vi "Elevator Controller Code.vi"(5 "Cut Off Switch":bool, 6 "Bottom Switch":bool, 7 "Top Switch":bool, 8 "Down":bool, 9 "Up":bool, 10 "Decrease":bool, 11 "Increase":bool) -> (1 "Tote Offset":dbl, 3 "Motor Value":dbl)   [LabVIEW 2014]
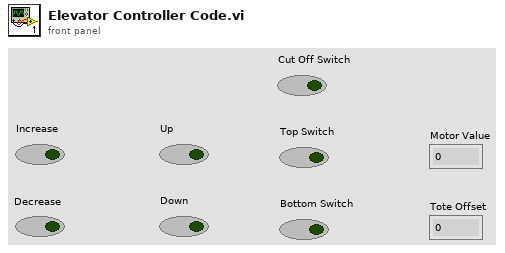
[diagram p1: front panel]
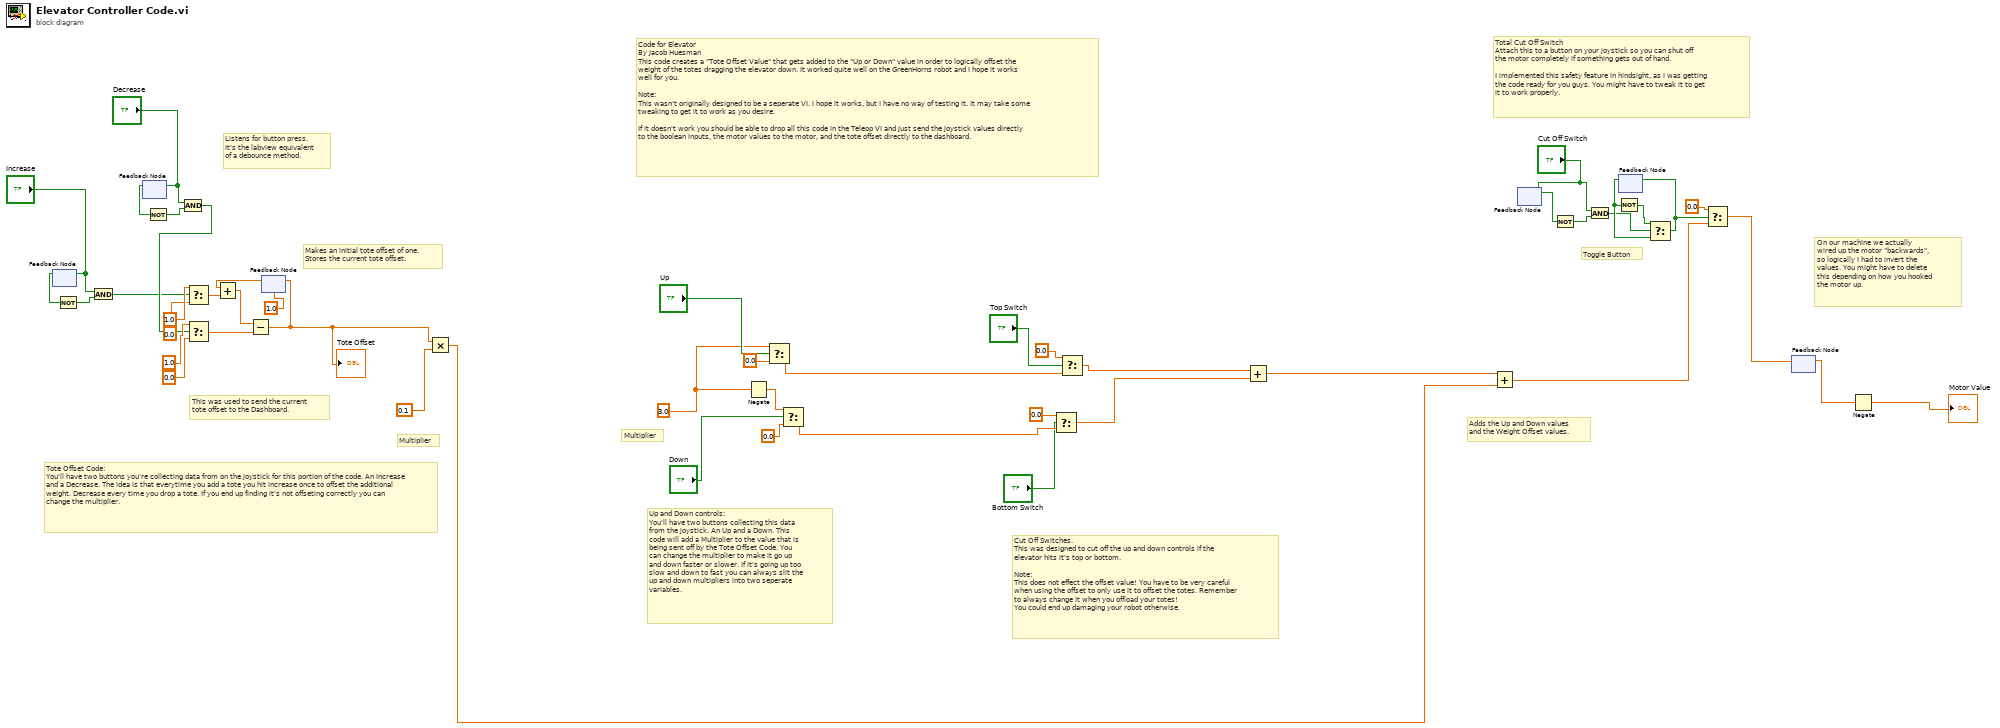
[diagram p0: block diagram]
diagram:
  w18 = 3.0
  # "Toggle Button"
  # "Total Cut Off Switch\nAttach this to a button on your joystick so you can shut off\nthe motor completely if something gets out of hand.\n\nI implemented this safety feature in hindsight, as I was getting\nthe code ready for you guys. You might have to tweak it to get \nit to work properly."
  # "Cut Off Switches.\nThis was designed to cut off the up and down controls if the\nelevator hits it's top or bottom.\n\nNote:\nThis does not effect the offset value! You have to be very careful\nwhen using the offset to only use it to offset the totes. Remember\nto always change it when you offload your totes! \nYou could end up damaging your robot otherwise."
  # "On our machine we actually\nwired up the motor \"backwards\",\nso logically I had to invert the\nvalues. You might have to delete\nthis depending on how you hooked\nthe motor up."
  # "Adds the Up and Down values\nand the Weight Offset values."
  # "Makes an initial tote offset of one.\nStores the current tote offset."
  # "Listens for button press.\nIt's the labview equivalent\nof a debounce method."
  # "This was used to send the current \ntote offset to the Dashboard."
  # "Multiplier"
  # "Up and Down controls:\nYou'll have two buttons collecting this data\nfrom the joystick. An Up and a Down. This \ncode will add a Multiplier to the value that is\nbeing sent off by the Tote Offset Code. You\ncan change the multiplier to make it go up\nand down faster or slower. If it's going up too\nslow and down to fast you can always slit the\nup and down multipliers into two seperate \nvariables."
  # "Multiplier"
  # "Tote Offset Code:\nYou'll have two buttons you're collecting data from on the joystick for this portion of the code. An Increase and a Decrease. The idea is that everytime you add a tote you hit increase once to offset the additional weight. Decrease every time you drop a tote. If you end up finding it's not offseting correctly you can change the multiplier."
  # "Code for Elevator\nBy Jacob Huesman\nThis code creates a \"Tote Offset Value\" that gets added to the \"Up or Down\" value in order to logically offset the\nweight of the totes dragging the elevator down. It worked quite well on the GreenHorns robot and I hope it works\nwell for you.\n\nNote:\nThis wasn't originally designed to be a seperate VI. I hope it works, but I have no way of testing it. It may take some\ntweaking to get it to work as you desire. \n\nIf it doesn't work you should be able to drop all this code in the Teleop VI and just send the joystick values directly\nto the boolean inputs, the motor values to the motor, and the tote offset directly to the dashboard."
  n1 = feedback #1() -> (w33:bool)  [unwired: 1 in]
  n2 = feedback-in #1("Increase") -> ()
  n3 = Not(x=w33) -> (.not. x?=w34:bool)
  n4 = And(x="Increase", y=w34) -> (x .and. y?=w32:bool)
  n5 = feedback #2() -> (w36:bool)  [unwired: 1 in]
  n6 = feedback-in #2("Decrease") -> ()
  n7 = Not(x=w36) -> (.not. x?=w37:bool)
  n8 = And(x="Decrease", y=w37) -> (x .and. y?=w35:bool)
  n9 = Select(t=1.0, s=w32, f=0.0) -> (s? t:f=w41:dbl)
  n10 = Select(t=1.0, s=w35, f=0.0) -> (s? t:f=w39:dbl)
  n11 = feedback #3(1.0 ("f")) -> (w40:dbl)
  n12 = Add(x=w40, y=w41) -> (x+y=w38:dbl)
  n13 = Subtract(x=w38, y=w39) -> (x-y=w15:dbl)
  "Tote Offset" <- w15
  n14 = feedback-in #3(w15) -> ()
  n15 = Multiply(x=w15, y=0.1) -> (x*y=w28:dbl)
  n16 = Negate(x=w18) -> (-x=w29:dbl)
  n17 = Select(t=w18, s="Up", f=0.0) -> (s? t:f=w47:dbl)
  n18 = Select(t=w29, s="Down", f=0.0) -> (s? t:f=w24:dbl)
  n19 = Select(t=0.0, s="Bottom Switch", f=w24) -> (s? t:f=w25:dbl)
  n20 = Select(t=0.0, s="Top Switch", f=w47) -> (s? t:f=w27:dbl)
  n21 = Add(x=w27, y=w25) -> (x+y=w16:dbl)
  n22 = Add(x=w16, y=w28) -> (x+y=w9:dbl)
  n23 = feedback #4() -> (w3:bool)  [unwired: 1 in]
  n24 = feedback-in #4("Cut Off Switch") -> ()
  n25 = Not(x=w3) -> (.not. x?=w4:bool)
  n26 = And(x="Cut Off Switch", y=w4) -> (x .and. y?=w5:bool)
  n27 = feedback #5() -> (w6:bool)  [unwired: 1 in]
  n28 = Not(x=w6) -> (.not. x?=w7:bool)
  n29 = Select(t=w7, s=w5, f=w6) -> (s? t:f=w1:bool)
  n30 = feedback-in #5(w1) -> ()
  n31 = Select(t=0.0, s=w1, f=w9) -> (s? t:f=w10:dbl)
  n32 = feedback-in #6(w10) -> ()
  n33 = feedback #6() -> (w8:dbl)  [unwired: 1 in]
  n34 = Negate(x=w8) -> (-x=→"Motor Value":dbl)
